vi "Items.vi"(8 "error in (no error)":errorcluster, 11 "BufferedArray in":refnum<class "BufferedArray.lvclass">) -> (0 "error out":errorcluster, 1 "Items":refnum<class>[](array[class]), 3 "BufferedArray out":refnum<class "BufferedArray.lvclass">)   [LabVIEW 2013, in "LapDog.Collections.v_.Lists.Implementations.lvlib" / "BufferedArray.lvclass"]
doc: "Returns a copy of all the elements in the list."
uses:
  BufferedArray.lvclass
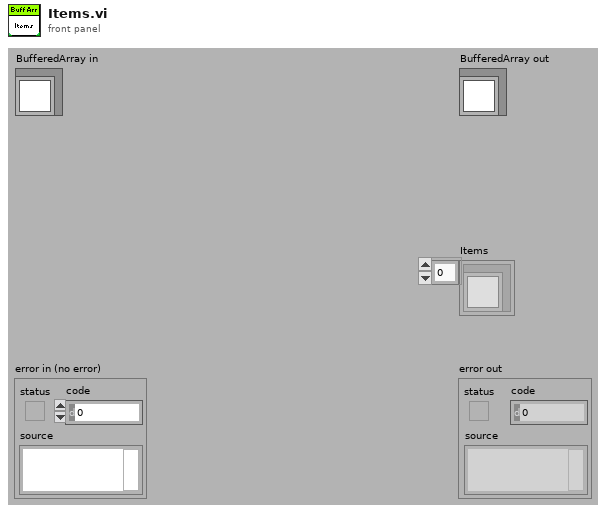
[diagram p1: front panel]
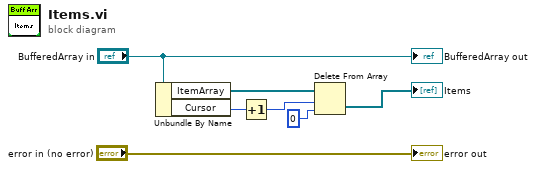
[diagram p0: block diagram]
diagram:
  n1 = Unbundle By Name("BufferedArray in") -> ("ItemArray"=w5:refnum<class>[], "Cursor"=w4:i32)
  n2 = Increment(x=w4) -> (x+1=w1:i32)
  n3 = Delete From Array(array=w5, length=w1, index=0) -> (deleted portion=→"Items":refnum<class>[])  [unwired: 1 out]
  "error out" <- "error in (no error)"
  "BufferedArray out" <- "BufferedArray in"
